vi "Get Pressure Readings.vi"(8 "error in (no error)":errorcluster) -> (0 "error out":errorcluster, 2 "Leak Rate":dbl, 3 "NI-DAQ Pressure":dbl, 5 "Instantaneous":dbl)   [LabVIEW 2015]
uses:
  Common/Buffers/Snapshot/Snapshot.lvclass
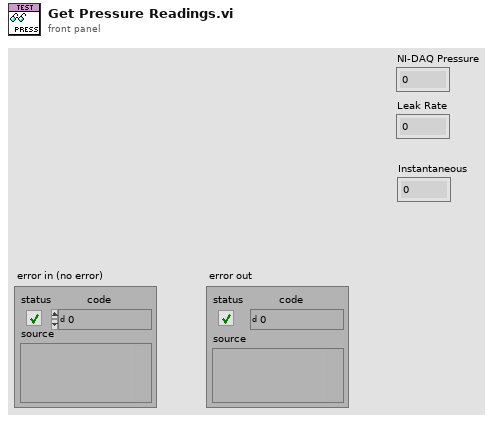
[diagram p1: front panel]
types:
  T1 = typedef "Snapshot.lvclass/Session Handle.ctl" = refnum<data-value>
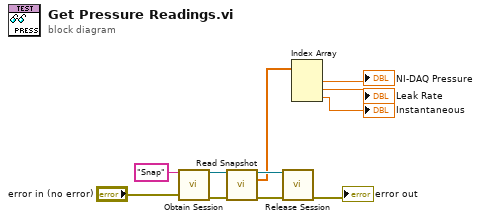
[diagram p0: block diagram]
diagram:
  n1 = call "Obtain Session.vi"("Session  Name ()"="Snap", "error in (no error)"="error in (no error)") -> ("Session Handle"=w8:T1, "error out"=w9:errorcluster)  [unwired: 12 in]
  n2 = call "Read Snapshot.vi"("Session Handle in"=w8, "error in (no error)"=w9) -> ("Session Handle out"=w6:T1, "Buffer"=w4:dbl[], "error out"=w7:errorcluster)  [unwired: 11 in]
  n3 = call "Release Session.vi"("Session Handle"=w6, "error in (no error)"=w7) -> ("error out"=→"error out":errorcluster)  [unwired: 13 in]
  n4 = Index Array(array=w4) -> (element #1=→"NI-DAQ Pressure":dbl, element #2=→"Leak Rate":dbl, element #3=→"Instantaneous":dbl)  [unwired: 3 in]
